vi "Post Post Build Action.vi"() -> (0 "error out":errorcluster)   [LabVIEW 2020]
uses:
  0ded7f5a-f2f5-45de-b494-e0b69212a52f.vi
panel:
  out "vilib binaries":path
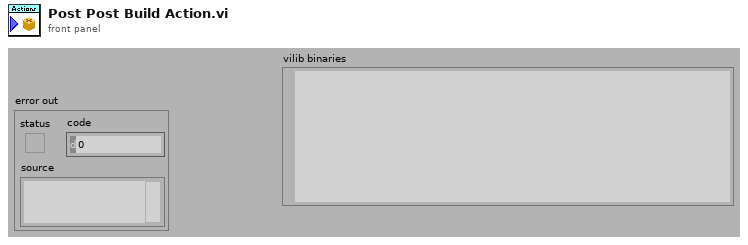
[diagram p1: front panel]
types:
  T1 = cluster{"Source Dist":path, "Zip Location":path, "vi.lib location":path, "Binaries Dir":path, "Binaries Wildcard Name":path}
  T2 = enum16{"Build Paths", "Remark Items to Exclude Compiled Code", "Rewild CLFNs for Zip", "Create Zip File", "Move Binaries to VI lib"}
  T3 = enum16{"Build Paths", "Remark Items to Exclude Compiled Code", "Rewild CLFNs for Zip", "Create Zip File", "Move Binaries to VI lib"}[]
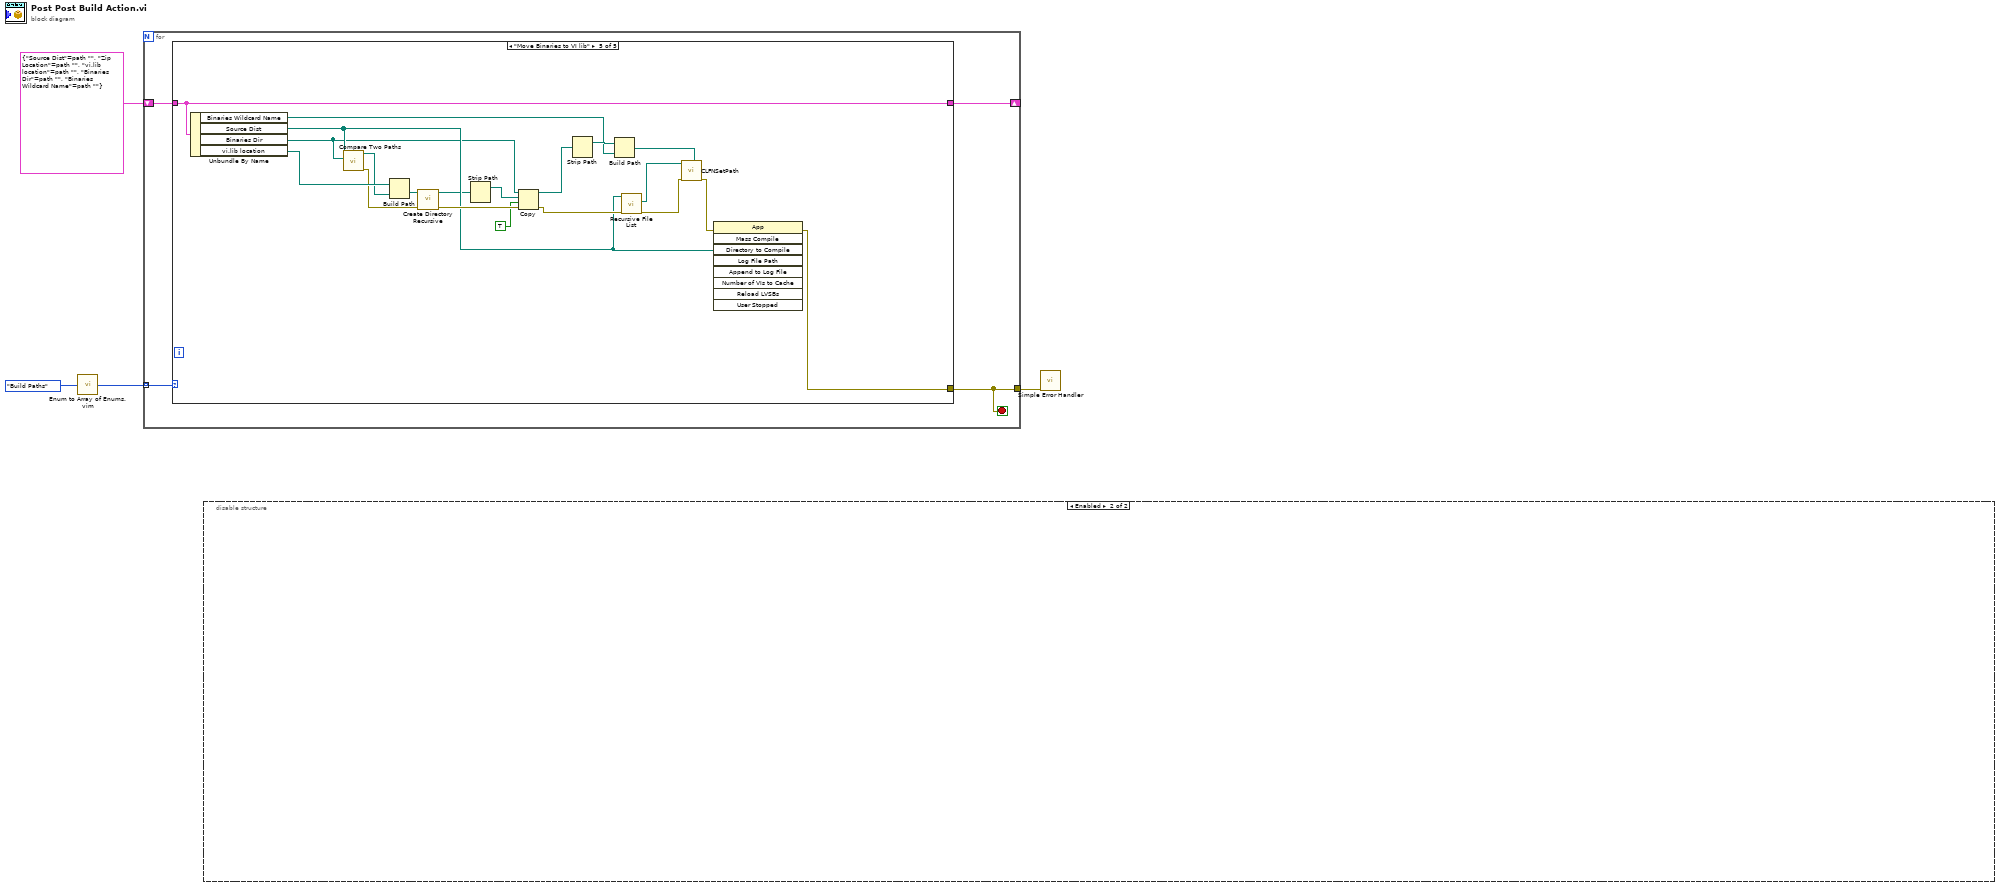
[diagram p0: block diagram]
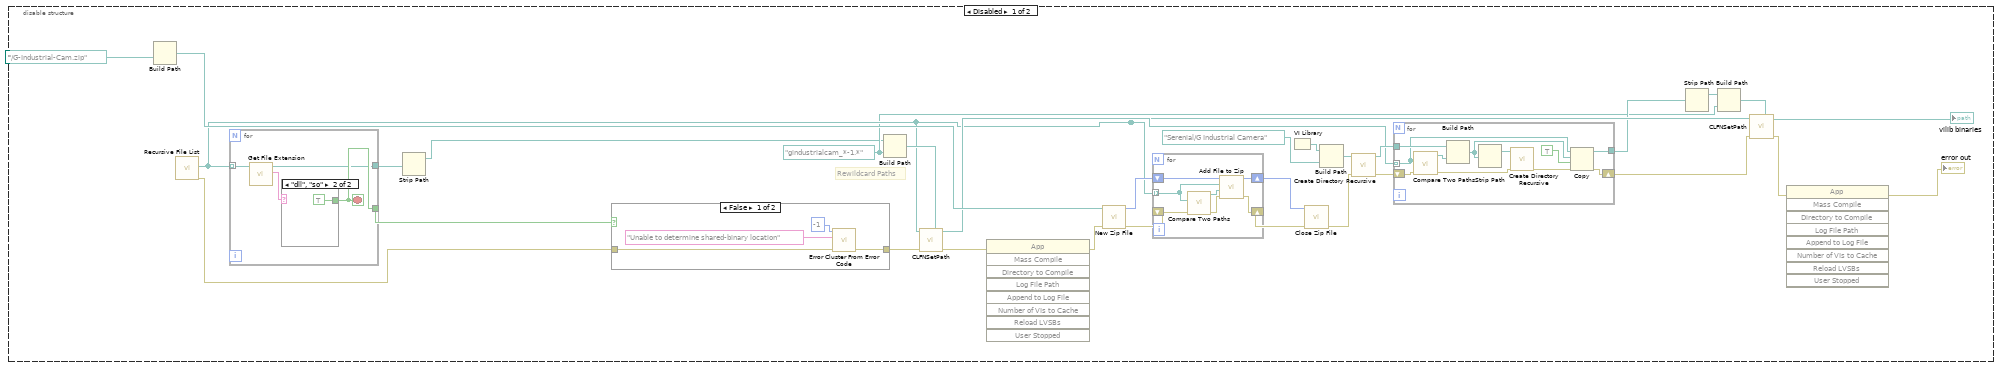
[diagram p2: hidden frame]
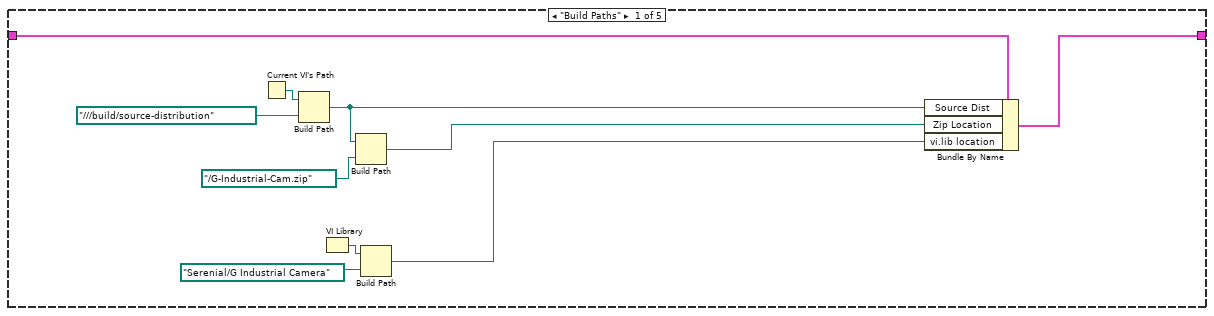
[diagram p5: hidden frame]
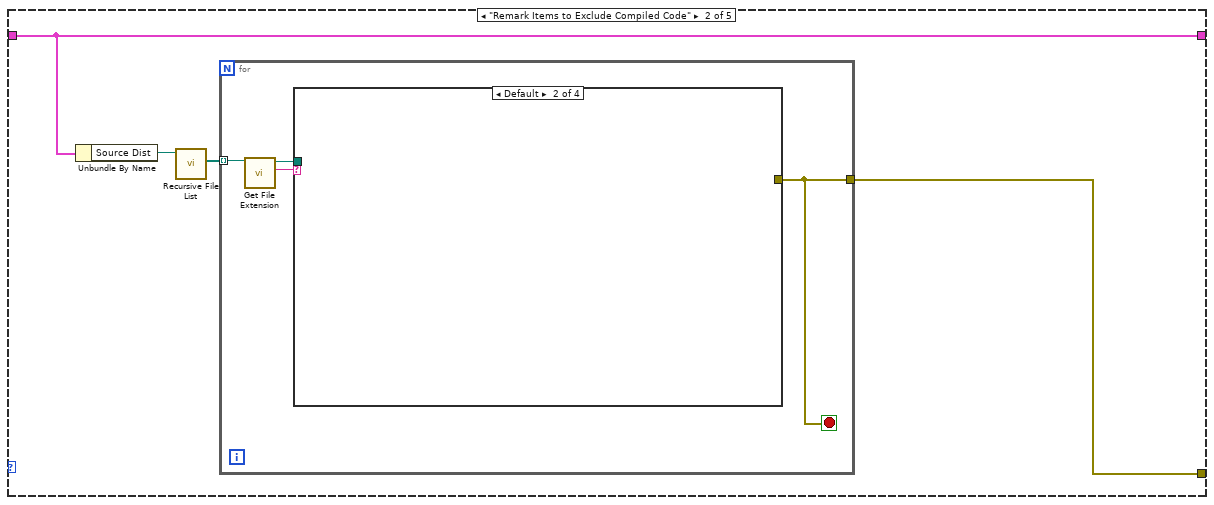
[diagram p6: hidden frame]
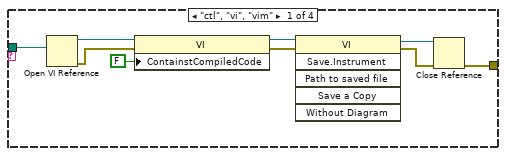
[diagram p7: hidden frame]
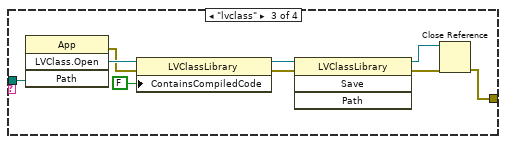
[diagram p8: hidden frame]
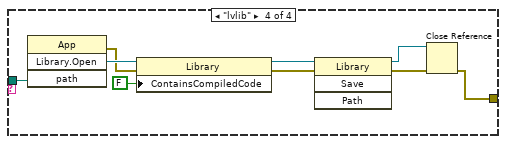
[diagram p9: hidden frame]
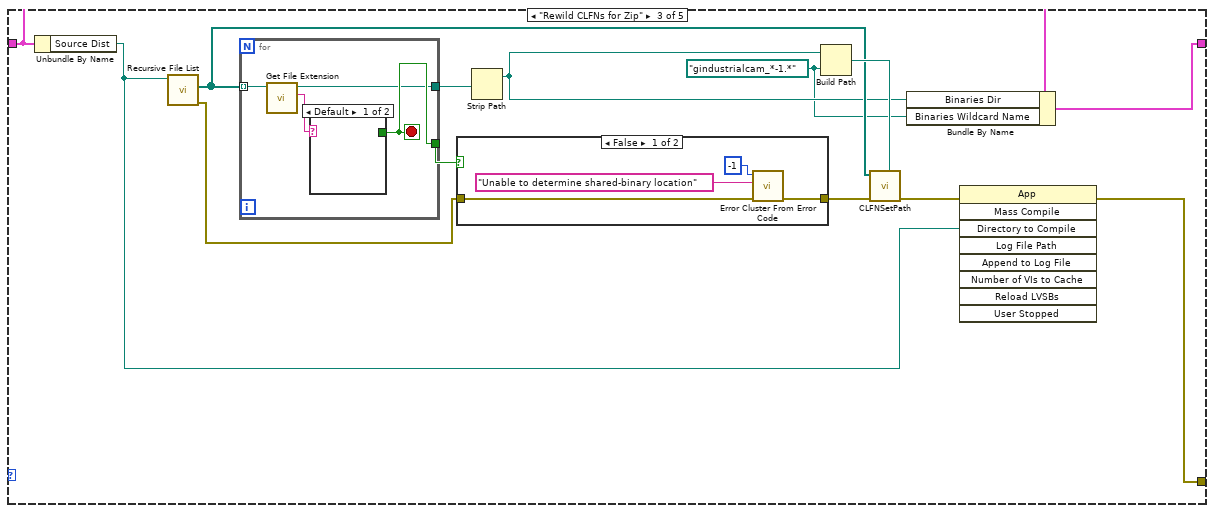
[diagram p10: hidden frame]
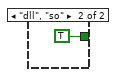
[diagram p12: hidden frame]
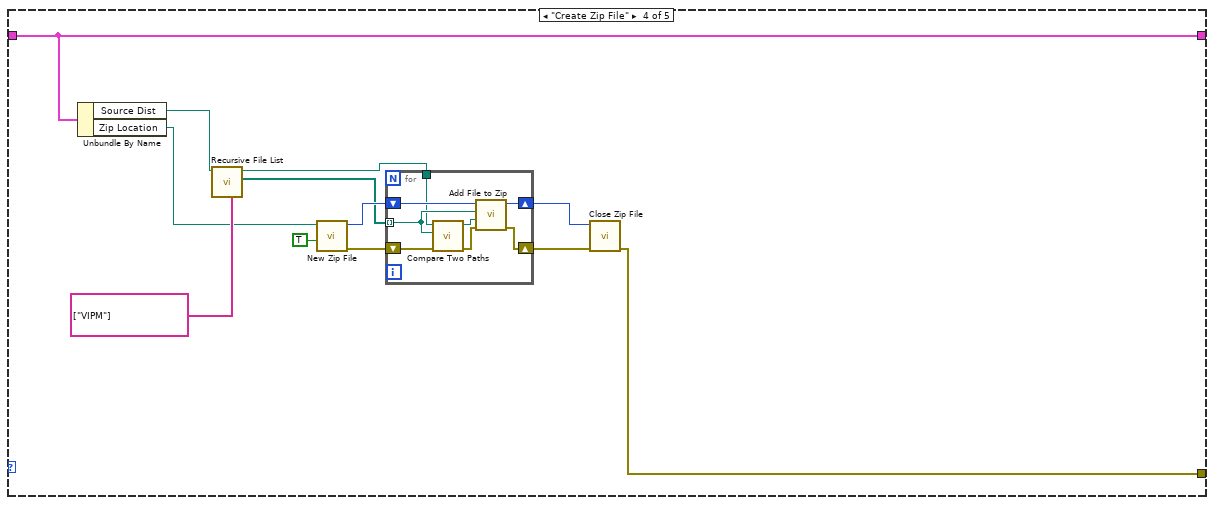
[diagram p13: hidden frame]
diagram:
  n1 = call "Enum to Array of Enums.vim"("enum"=T2."Build Paths") -> ("array of enums"=w2:T3)
  n2 = for {
    shift-right: [w6] -> _
    shift-left: T1 {"Source Dist"=path "", "Zip Location"=path "", "vi.lib location"=path "", "Binaries Dir"=path "", "Binaries Wildcard Name"=path ""} -> [w7]
    tunnel: w2 -> [w8] mode=indexing
    tunnel: [w5] -> w1
    stop <- w5 stop-if-true
    n3 = case shown="\"Move Binaries to VI lib\"" w8 {
      tunnel: w7 -> [w18 w22 w59 w84 w116]
      tunnel: [w9 w22 w56 w84 w116] -> w6
      tunnel: [_ w19 w58 w78 w107] -> w5
      frame "Build Paths" {
        n4 = Current VI's Path() -> (path=w17:path)
        n5 = Build Path(base path=w17, name or relative path=path "../../../build/source-distribution") -> (appended path=w14:path)
        n6 = VI Library() -> (path=w12:path)
        n7 = Build Path(base path=w14, name or relative path=path "../G-Industrial-Cam.zip") -> (appended path=w13:path)
        n8 = Build Path(base path=w12, name or relative path=path "Serenial/G Industrial Camera") -> (appended path=w10:path)
        n9 = Bundle By Name(cluster=w18, "Source Dist"=w14, "Zip Location"=w13, "vi.lib location"=w10) -> (w9:T1)
      }
      frame "Remark Items to Exclude Compiled Code" {
        n10 = Unbundle By Name(w22) -> ("Source Dist"=w21:path)
        n11 = call <vilib>:"Recursive File List.vi"("Folder Path"=w21) -> ("All Files in Dir"=w20:path[])  [unwired: 6 in, 4 out]
        n12 = for {
          tunnel: w20 -> [w26] mode=indexing
          tunnel: [w23] -> w19
          stop <- w23 stop-if-true
          n13 = call <vilib>:"Get File Extension.vi"("file"=w26) -> ("lowercase file extension"=w25:string, "dup file"=w24:path)  [unwired: 6 in, 3 out]
          n14 = case shown="Default" w25 {
            tunnel: w24 -> [w35 _ w44 w53]
            tunnel: [w30 _ w37 w45] -> w23
            frame "ctl", "vi", "vim" {
              n15 = Open VI Reference(vi path=w35) -> (vi reference=w34:refnum<vi>, error out=w33:errorcluster)  [unwired: 5 in]
              n16 = property class="VI"(reference=w34, error in=w33, "ContainstCompiledCode"=FALSE ("Contains Compiled Code")) -> (reference out=w28:refnum<vi>, error out=w31:errorcluster)
              n17 = invoke class="VI" method="Save.Instrument"(reference=w28, error in=w31) -> (reference out=w27:refnum<vi>, error out=w29:errorcluster)  [unwired: 4 in, 4 out]
              n18 = Close Reference(reference=w27, error in (no error)=w29) -> (error out=w30:errorcluster)
            }
            frame Default {
            }
            frame "lvclass" {
              n19 = invoke class="App" method="LVClass.Open"("Path"=w44) -> (error out=w41:errorcluster, "LVClass.Open"=w43:refnum<vi>)  [unwired: 3 in, 2 out]
              n20 = property class="LVClassLibrary"(reference=w43, error in=w41, "ContainsCompiledCode"=FALSE ("Contains Compiled Code")) -> (reference out=w40:refnum<vi>, error out=w39:errorcluster)
              n21 = invoke class="LVClassLibrary" method="Save"(reference=w40, error in=w39) -> (reference out=w36:refnum<vi>, error out=w38:errorcluster)  [unwired: 2 in, 2 out]
              n22 = Close Reference(reference=w36, error in (no error)=w38) -> (error out=w37:errorcluster)
            }
            frame "lvlib" {
              n23 = invoke class="App" method="Library.Open"("path"=w53) -> (error out=w50:errorcluster, "Open Library"=w52:refnum<vi>)  [unwired: 3 in, 2 out]
              n24 = property class="Library"(reference=w52, error in=w50, "ContainsCompiledCode"=FALSE ("Contains Compiled Code")) -> (reference out=w49:refnum<vi>, error out=w48:errorcluster)
              n25 = invoke class="Library" method="Save"(reference=w49, error in=w48) -> (reference out=w46:refnum<vi>, error out=w47:errorcluster)  [unwired: 2 in, 2 out]
              n26 = Close Reference(reference=w46, error in (no error)=w47) -> (error out=w45:errorcluster)
            }
          }
        }
      }
      frame "Rewild CLFNs for Zip" {
        w54 = path "gindustrialcam_*-1.*" ("New Path")
        n27 = Unbundle By Name(w59) -> ("Source Dist"=w57:path)
        n28 = call <vilib>:"Recursive File List.vi"("Folder Path"=w57) -> ("error out"=w62:errorcluster, "All Files in Dir"=w61:path[])  [unwired: 6 in, 3 out]
        n29 = for {
          tunnel: w61 -> [w75] mode=indexing
          tunnel: [w73] -> w66
          tunnel: [w72] -> w60
          stop <- w73 stop-if-true
          n30 = call <vilib>:"Get File Extension.vi"("file"=w75) -> ("lowercase file extension"=w74:string, "dup file"=w72:path)  [unwired: 6 in, 3 out]
          n31 = case shown="Default" w74 {
            tunnel: [_ TRUE] -> w73
            frame Default {
            }
            frame "dll", "so" {
            }
          }
        }
        n32 = case shown="False" w66 {
          tunnel: [w70 w71] -> w65
          tunnel: w62 -> [w67 w71]
          frame False {
            n33 = call <vilib>:"Error Cluster From Error Code.vi"("error in (no error)"=w67, "error message (\"\")"="Unable to determine shared-binary location" ("error message (\"\")"), "error code (0)"=-1) -> ("error out"=w70:errorcluster)  [unwired: 6 in]
          }
          frame True {
          }
        }
        n34 = Strip Path(path=w60) -> (stripped path=w55:path)  [unwired: 1 out]
        n35 = Build Path(base path=w55, name or relative path=w54) -> (appended path=w64:path)
        n36 = call "CLFNSetPath.vi"("New Path"=w64, "error in (no error)"=w65, "Files"=w61) -> ("error out"=w63:errorcluster)  [unwired: 7 in, 1 out]
        n37 = Bundle By Name(cluster=w59, "Binaries Dir"=w55, "Binaries Wildcard Name"=w54) -> (w56:T1)
        n38 = invoke class="App" method="Mass Compile"(error in=w63, "Directory to Compile"=w57) -> (error out=w58:errorcluster)  [unwired: 7 in, 8 out]
      }
      frame "Create Zip File" {
        n39 = Unbundle By Name(w84) -> ("Source Dist"=w83:path, "Zip Location"=w77:path)
        n40 = call <vilib>:"Recursive File List.vi"("Folders to Exclude"=string[] ["VIPM"], "Folder Path"=w83) -> ("All Files in Dir"=w81:path[], "dup Folder Path"=w80:path)  [unwired: 5 in, 3 out]
        n41 = call <vilib>:"New Zip File.vi"("confirm overwrite? (F)"=TRUE, "target"=w77) -> ("error out"=w87:errorcluster, "zip file out"=w88:i64)  [unwired: 3 in, 1 out]
        n42 = for {
          tunnel: w81 -> [w92] mode=indexing
          shift-right: [w91] -> w86
          shift-left: w88 -> [w96]
          shift-right: [w90] -> w85
          shift-left: w87 -> [w94]
          tunnel: w80 -> [w89]
          n43 = call <vilib>:"Compare Two Paths.vi"("error in (no error)"=w94, "Path 2"=w92, "Path 1"=w89) -> ("error out"=w93:errorcluster, "Relative Path from 1 to 2"=w95:path)  [unwired: 5 in, 2 out]
          n44 = call <vilib>:"Add File to Zip.vi"("error in (no error)"=w93, "destination path in zip"=w95, "source file path"=w92, "zip file in"=w96) -> ("error out"=w90:errorcluster, "zip file out"=w91:i64)  [unwired: 6 in]
        }
        n45 = call <vilib>:"Close Zip File.vi"("error in (no error)"=w85, "zip file in"=w86) -> ("error out"=w78:errorcluster)  [unwired: 5 in]
      }
      frame "Move Binaries to VI lib" {
        n46 = Unbundle By Name(w116) -> ("Binaries Wildcard Name"=w110:path, "Source Dist"=w105:path, "Binaries Dir"=w101:path, "vi.lib location"=w104:path)
        n47 = call <vilib>:"Compare Two Paths.vi"("Path 2"=w101, "Path 1"=w105) -> ("error out"=w98:errorcluster, "Relative Path from 1 to 2"=w102:path)  [unwired: 6 in, 2 out]
        n48 = Build Path(base path=w104, name or relative path=w102) -> (appended path=w103:path)
        n49 = call <vilib>:"Create Directory Recursive.vi"("error in (no error)"=w98, "directory"=w103) -> ("error out"=w106:errorcluster, "directory copy"=w100:path)  [unwired: 3 in, 1 out]
        n50 = Strip Path(path=w100) -> (stripped path=w97:path)  [unwired: 1 out]
        n51 = Copy(8:w106, 9:TRUE ("overwrite (F)"), 10:w97, 11:w101) -> (0:w112:errorcluster, 3:w111:path)  [unwired: 1 in, 1 out]
        n52 = Strip Path(path=w111) -> (stripped path=w115:path)  [unwired: 1 out]
        n53 = Build Path(base path=w115, name or relative path=w110) -> (appended path=w114:path)
        n54 = call <vilib>:"Recursive File List.vi"("error in (no error)"=w112, "Folder Path"=w105) -> ("error out"=w109:errorcluster, "All Files in Dir"=w108:path[])  [unwired: 5 in, 3 out]
        n55 = call "CLFNSetPath.vi"("New Path"=w114, "error in (no error)"=w109, "Files"=w108) -> ("error out"=w113:errorcluster)  [unwired: 7 in, 1 out]
        n56 = invoke class="App" method="Mass Compile"(error in=w113, "Directory to Compile"=w105) -> (error out=w107:errorcluster)  [unwired: 7 in, 8 out]
      }
    }
  }
  n57 = disable-structure shown="Enabled" {
    frame Disabled {
      w121 = path "gindustrialcam_*-1.*" ("New Path")
      # "Rewildcard Paths"
      n58 = Build Path(name or relative path=path "../G-Industrial-Cam.zip") -> (appended path=w139:path)  [unwired: 1 in]
      n59 = call <vilib>:"Recursive File List.vi"() -> ("error out"=w127:errorcluster, "All Files in Dir"=w125:path[])  [unwired: 7 in, 3 out]
      n60 = for {
        tunnel: w125 -> [w172] mode=indexing
        tunnel: [w170] -> w145
        tunnel: [w169] -> w120
        stop <- w170 stop-if-true
        n61 = call <vilib>:"Get File Extension.vi"("file"=w172) -> ("lowercase file extension"=w171:string, "dup file"=w169:path)  [unwired: 6 in, 3 out]
        n62 = case shown="\"dll\", \"so\"" w171 {
          tunnel: [_ TRUE] -> w170
          frame Default {
          }
          frame "dll", "so" {
          }
        }
      }
      n63 = Strip Path(path=w120) -> (stripped path=w119:path)  [unwired: 1 out]
      n64 = case shown="False" w145 {
        tunnel: [w167 w168] -> w144
        tunnel: w127 -> [w164 w168]
        frame False {
          n65 = call <vilib>:"Error Cluster From Error Code.vi"("error in (no error)"=w164, "error message (\"\")"="Unable to determine shared-binary location" ("error message (\"\")"), "error code (0)"=-1) -> ("error out"=w167:errorcluster)  [unwired: 6 in]
        }
        frame True {
        }
      }
      n66 = Build Path(base path=w119, name or relative path=w121) -> (appended path=w143:path)
      n67 = call "CLFNSetPath.vi"("New Path"=w143, "error in (no error)"=w144, "Files"=w125) -> ("error out"=w142:errorcluster, "Shared Binaries"=w128:path[])  [unwired: 7 in]
      n68 = invoke class="App" method="Mass Compile"(error in=w142) -> (error out=w141:errorcluster)  [unwired: 8 in, 8 out]
      n69 = call <vilib>:"New Zip File.vi"("error in (no error)"=w141, "target"=w139) -> ("error out"=w137:errorcluster, "zip file out"=w138:i64)  [unwired: 3 in, 1 out]
      n70 = for {
        tunnel: w125 -> [w159] mode=indexing
        shift-right: [w158] -> w136
        shift-left: w138 -> [w163]
        shift-right: [w157] -> w135
        shift-left: w137 -> [w161]
        n71 = call <vilib>:"Compare Two Paths.vi"("error in (no error)"=w161, "Path 2"=w159) -> ("error out"=w160:errorcluster, "Relative Path from 1 to 2"=w162:path)  [unwired: 6 in, 2 out]
        n72 = call <vilib>:"Add File to Zip.vi"("error in (no error)"=w160, "destination path in zip"=w162, "source file path"=w159, "zip file in"=w163) -> ("error out"=w157:errorcluster, "zip file out"=w158:i64)  [unwired: 6 in]
      }
      n73 = VI Library() -> (path=w134:path)
      n74 = call <vilib>:"Close Zip File.vi"("error in (no error)"=w135, "zip file in"=w136) -> ("error out"=w131:errorcluster)  [unwired: 5 in]
      n75 = Build Path(base path=w134, name or relative path=path "Serenial/G Industrial Camera") -> (appended path=w132:path)
      n76 = call <vilib>:"Create Directory Recursive.vi"("error in (no error)"=w131, "directory"=w132) -> ("error out"=w129:errorcluster, "directory copy"=w130:path)  [unwired: 3 in, 1 out]
      n77 = for {
        tunnel: w130 -> [w156]
        tunnel: w128 -> [w153] mode=indexing
        shift-right: [w151] -> w126
        shift-left: w129 -> [w154]
        tunnel: [w146] -> w124
        n78 = call <vilib>:"Compare Two Paths.vi"("error in (no error)"=w154, "Path 2"=w153) -> ("error out"=w152:errorcluster, "Relative Path from 1 to 2"=w155:path)  [unwired: 6 in, 2 out]
        n79 = Build Path(base path=w156, name or relative path=w155) -> (appended path=w148:path)
        n80 = Strip Path(path=w148) -> (stripped path=w149:path)  [unwired: 1 out]
        n81 = call <vilib>:"Create Directory Recursive.vi"("error in (no error)"=w152, "directory"=w149) -> ("error out"=w150:errorcluster)  [unwired: 3 in, 2 out]
        n82 = Copy(8:w150, 9:TRUE ("overwrite (F)"), 10:w148, 11:w153) -> (0:w151:errorcluster, 3:w146:path)  [unwired: 1 in, 1 out]
      }
      n83 = Strip Path(path=w124) -> (stripped path=w123:path)  [unwired: 1 out]
      n84 = Build Path(base path=w123, name or relative path=w121) -> (appended path=w122:path)
      "vilib binaries" <- w122
      n85 = call "CLFNSetPath.vi"("New Path"=w122, "error in (no error)"=w126, "Files"=w125) -> ("error out"=w118:errorcluster)  [unwired: 7 in, 1 out]
      n86 = invoke class="App" method="Mass Compile"(error in=w118) -> (error out=→"error out":errorcluster)  [unwired: 8 in, 8 out]
    }
    frame Enabled {
    }
  }
  n87 = call <vilib>:"Simple Error Handler.vi"("error in (no error)"=w1) -> ()  [unwired: 4 in, 5 out]
